vi "fgv_joystick.vi"(7 "cmd":enum16{"ini", "read", "close"}(ring), 8 "error in":errorcluster) -> (0 "error out":errorcluster, 2 "val":bool, 3 "joystick info-out":T1)   [LabVIEW 2021]
uses:
  Ctrl/cmd_common.ctl
  <vilib>/Utility/inputDevices.llb/joystickAcquire.vi
  <vilib>/Utility/inputDevices.llb/closeJoystick.vi
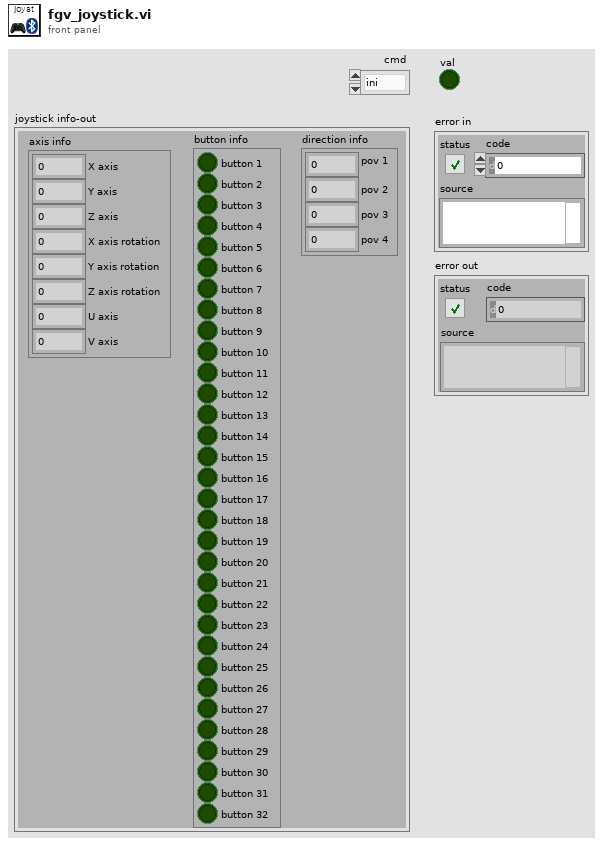
[diagram p1: front panel]
types:
  T1 = cluster{"axis info":cluster{"X axis":i32, "Y axis":i32, "Z axis":i32, "X axis rotation":i32, "Y axis rotation":i32, "Z axis rotation":i32, "U axis":i32, "V axis":i32}, "button info":cluster{"button 1":bool, "button 2":bool, "button 3":bool, "button 4":bool, "button 5":bool, "button 6":bool, "button 7":bool, "button 8":bool, "button 9":bool, "button 10":bool, "button 11":bool, "button 12":bool, "button 13":bool, "button 14":bool, "button 15":bool, "button 16":bool, "button 17":bool, "button 18":bool, "button 19":bool, "button 20":bool, "button 21":bool, "button 22":bool, "button 23":bool, "button 24":bool, "button 25":bool, "button 26":bool, "button 27":bool, "button 28":bool, "button 29":bool, "button 30":bool, "button 31":bool, "button 32":bool}, "direction info":cluster{"pov 1":i32, "pov 2":i32, "pov 3":i32, "pov 4":i32}}
  T2 = typedef "cmd_common.ctl" = enum16{"read", "write"}
  T3 = cluster{"X axis":i32, "Y axis":i32, "Z axis":i32, "X axis rotation":i32, "Y axis rotation":i32, "Z axis rotation":i32, "U axis":i32, "V axis":i32}
  T4 = cluster{"button 1":bool, "button 2":bool, "button 3":bool, "button 4":bool, "button 5":bool, "button 6":bool, "button 7":bool, "button 8":bool, "button 9":bool, "button 10":bool, "button 11":bool, "button 12":bool, "button 13":bool, "button 14":bool, "button 15":bool, "button 16":bool, "button 17":bool, "button 18":bool, "button 19":bool, "button 20":bool, "button 21":bool, "button 22":bool, "button 23":bool, "button 24":bool, "button 25":bool, "button 26":bool, "button 27":bool, "button 28":bool, "button 29":bool, "button 30":bool, "button 31":bool, "button 32":bool}
  T5 = cluster{"pov 1":i32, "pov 2":i32, "pov 3":i32, "pov 4":i32}
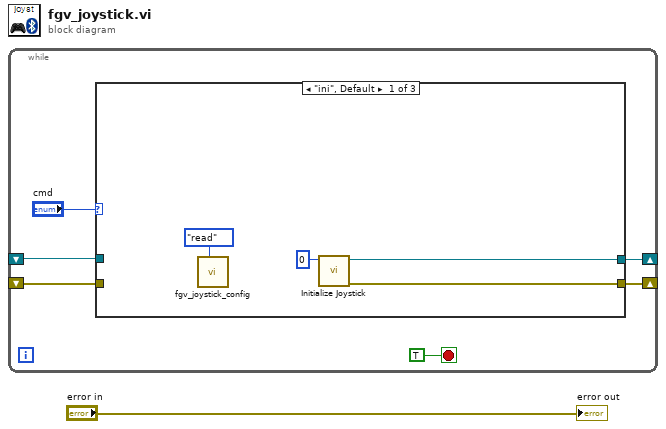
[diagram p0: block diagram]
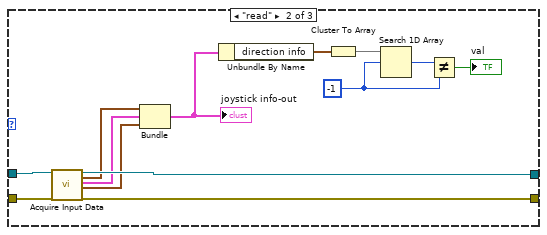
[diagram p2: hidden frame]
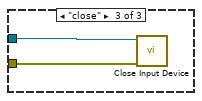
[diagram p3: hidden frame]
diagram:
  n1 = while {
    shift-right: [w5] -> _
    shift-left: _ -> [w3]
    shift-right: [w4] -> _
    shift-left: _ -> [w2]
    stop <- TRUE stop-if-true
    n2 = case shown="\"ini\", Default" "cmd" {
      tunnel: [w11 w24 _] -> w5
      tunnel: [w10 w23 _] -> w4
      tunnel: w3 -> [_ w22 w26]
      tunnel: w2 -> [_ w21 w25]
      frame "ini", Default {
        n3 = call "fgv_joystick_config.vi"("cmd"=cmd_common."read") -> ()  [unwired: 9 in, 2 out]
        n4 = call <vilib>:"Initialize Joystick.vi"("device index"=0) -> ("error out"=w10:errorcluster, "device ID"=w11:refnum<k1>)  [unwired: 9 in]
      }
      frame "read" {
        w17 = -1 ("element")
        n5 = call-poly <vilib>:"Acquire Input Data.vi"("device ID"=w22, "error in (no error)"=w21) -> ("device ID"=w24:refnum<k1>, "axis info"=w18:T3, "button info"=w19:T4, "direction info"=w20:T5, "error out"=w23:errorcluster)  [unwired: 13 in]
        n6 = Bundle("axis info"=w18, "button info"=w19, "direction info"=w20) -> (w13:T1)  [unwired: 1 in]
        "joystick info-out" <- w13
        n7 = Unbundle By Name(w13) -> ("direction info"=w14:T5)
        n8 = Cluster To Array(cluster=w14) -> (array=w15:i32[])
        n9 = Search 1D Array(1D array=w15, element=w17) -> (index of element=w16:i32)  [unwired: 1 in]
        n10 = Not Equal?(x=w16, y=w17) -> (x != y?=→"val":bool)
      }
      frame "close" {
        n11 = call-poly <vilib>:"Close Input Device.vi"("error in (no error)"=w25, "device ID"=w26) -> ()  [unwired: 8 in, 1 out]
      }
    }
  }
  "error out" <- "error in"
